vi "Define Global Constants.vi"   [LabVIEW 2014]
uses:
  Global Constants.vi
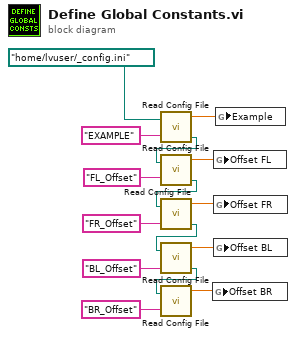
[diagram p0: block diagram]
diagram:
  n1 = call "Read Config File.vi"("file path"=path "/home/lvuser/_config.ini", "key"="EXAMPLE") -> ("value"=w5:dbl, "file path"=w13:path)  [unwired: 1 out]
  n2 = call "Read Config File.vi"("file path"=w13, "key"="FL_Offset") -> ("value"=w4:dbl, "file path"=w12:path)  [unwired: 1 out]
  n3 = call "Read Config File.vi"("file path"=w12, "key"="FR_Offset") -> ("value"=w3:dbl, "file path"=w11:path)  [unwired: 1 out]
  n4 = call "Read Config File.vi"("file path"=w11, "key"="BL_Offset") -> ("value"=w2:dbl, "file path"=w10:path)  [unwired: 1 out]
  n5 = call "Read Config File.vi"("file path"=w10, "key"="BR_Offset") -> ("value"=w1:dbl)  [unwired: 2 out]
  n6 = global write "Global Constants.vi" "Offset BR"(w1) -> ()
  n7 = global write "Global Constants.vi" "Offset FL"(w4) -> ()
  n8 = global write "Global Constants.vi" "Offset FR"(w3) -> ()
  n9 = global write "Global Constants.vi" "Offset BL"(w2) -> ()
  n10 = global write "Global Constants.vi" "Example"(w5) -> ()
